vi "Portcullis-CDF State Machine.vi"(0 "Collector Lift State":T1, 1 "Collect Lift Position":dbl, 2 "AutoLift Portcullis?":bool, 3 "AutoAdjust CDF?":bool, 4 "Keep at target?":bool, 5 "See Portcullis?":bool, 6 "See CDF?":bool, 8 "Collector Lift Man.  Request?":bool) -> (20 "Collector Lift State Out":T1)   [LabVIEW 2015]
uses:
  Typedefs/CollectorLiftStates.ctl
panel:
  in  "Thresh":dbl=1.0
  in  "CDF Set Up Position":dbl format="%#_13g"
  in  "Portcullis Set Up Position":dbl format="%#_13g"
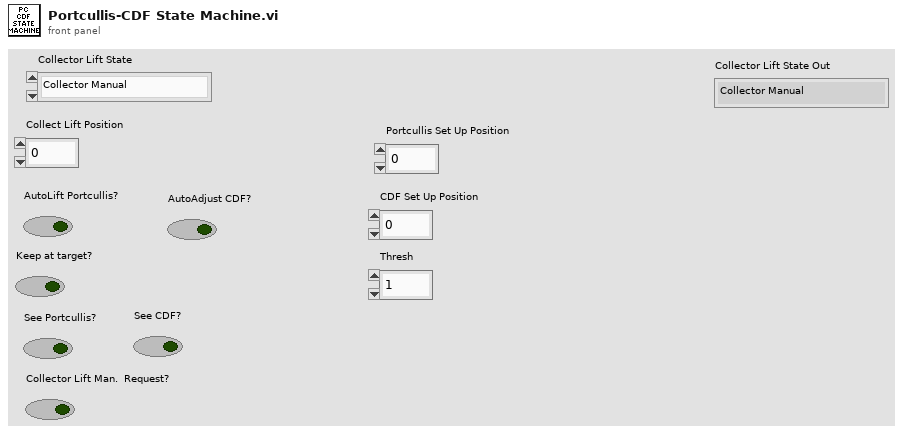
[diagram p1: front panel]
types:
  T1 = typedef "CollectorLiftStates.ctl" = enum16{"Collector Manual", "Stow", "Collect Position", "Spit Position", "Portcullis Set Up", "Portcullis Lift Up", "CDF Set Up", "Push CDF Down"}
  T2 = enum16{"Pass HMI Through Choice", "AutoAdjust CDF", "AutoLift PC"}
  T3 = enum16{"Go to set up ", "Keep at CDF", "Push Down CDF"}
  T4 = enum16{"Go to set up", "Keep At Portcullis", "Lift Up Portcullis"}
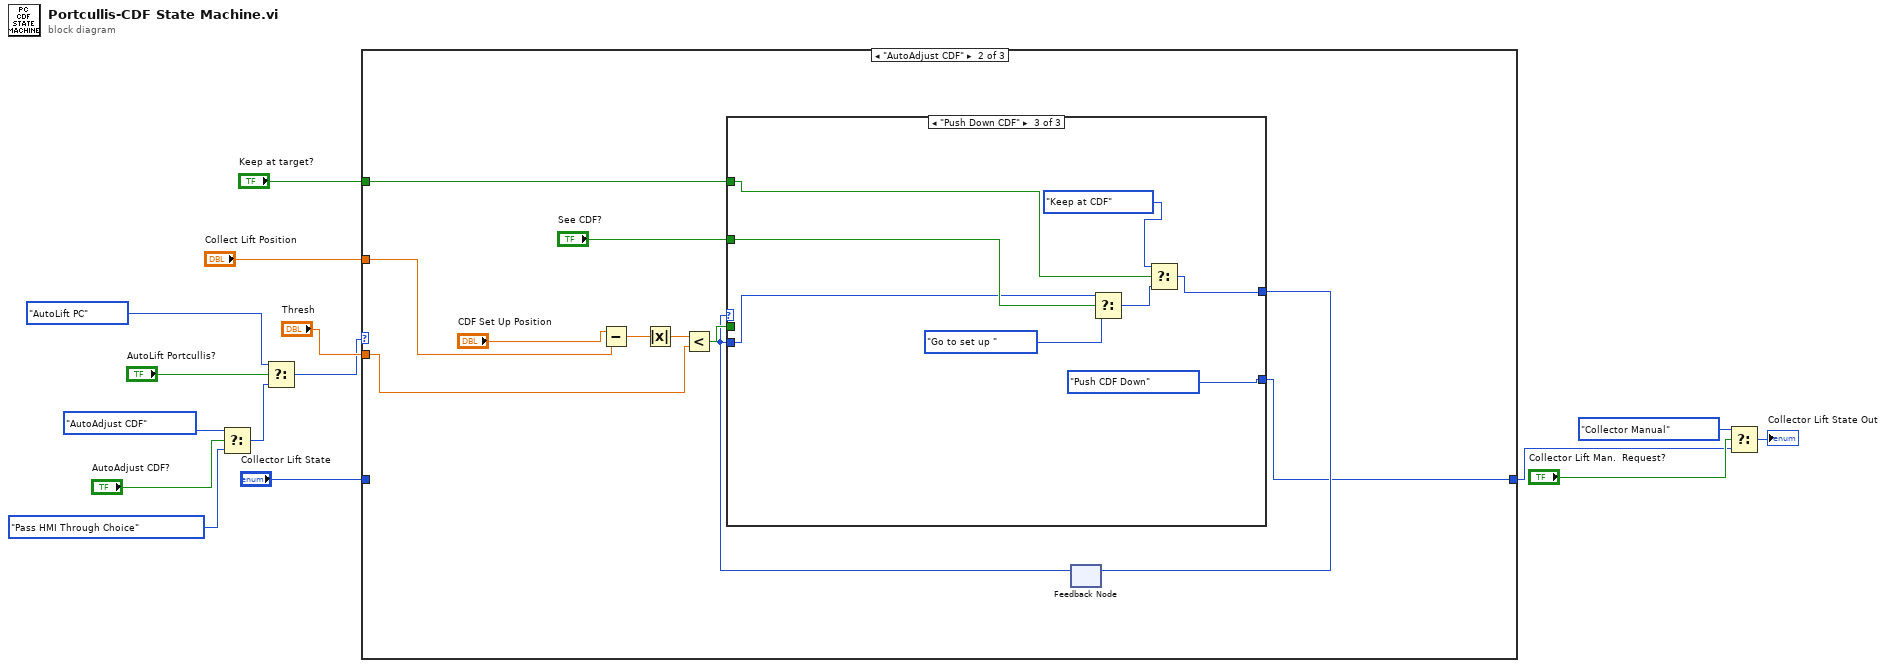
[diagram p0: block diagram]
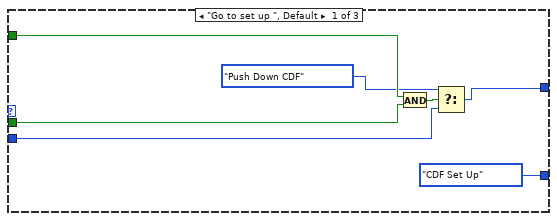
[diagram p3: hidden frame]
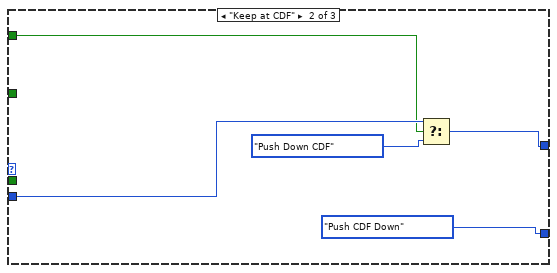
[diagram p4: hidden frame]
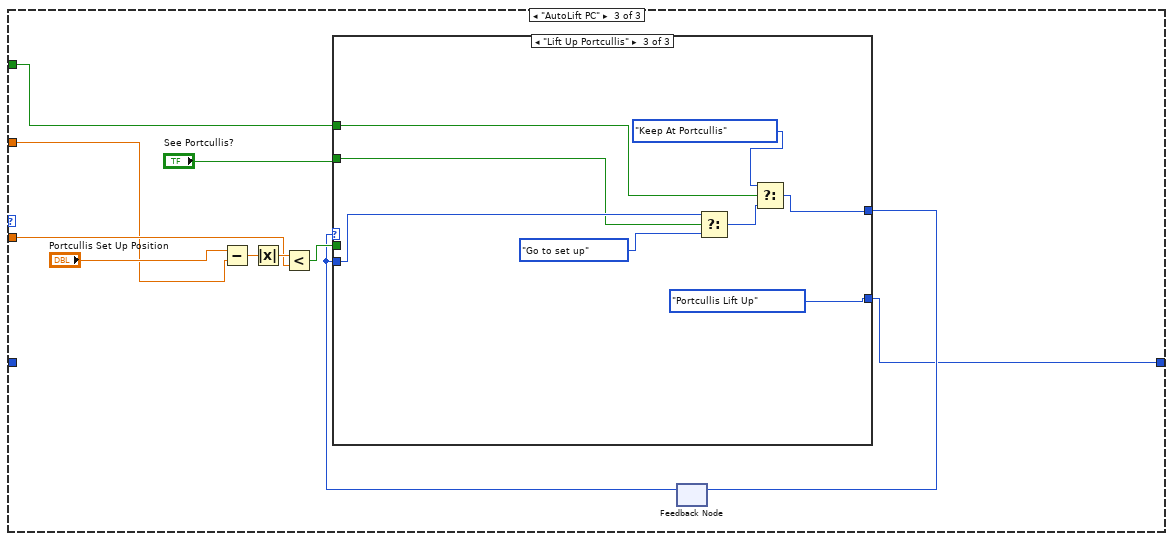
[diagram p5: hidden frame]
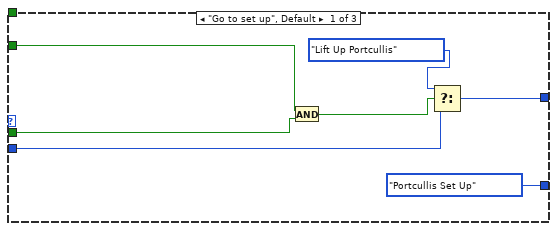
[diagram p6: hidden frame]
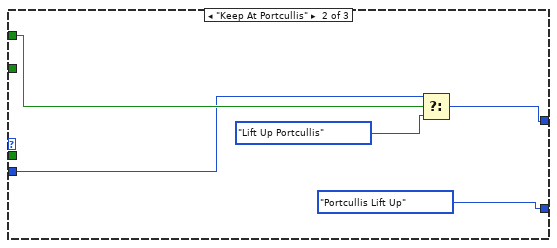
[diagram p7: hidden frame]
diagram:
  n1 = Select(t=T2."AutoAdjust CDF", s="AutoAdjust CDF?", f=T2."Pass HMI Through Choice") -> (s? t:f=w12:T2)
  n2 = Select(t=T2."AutoLift PC", s="AutoLift Portcullis?", f=w12) -> (s? t:f=w5:T2)
  n3 = case shown="\"AutoAdjust CDF\"" w5 {
    tunnel: [w16 w21 w52] -> w3
    tunnel: "Collector Lift State" -> [w16 _ _]
    tunnel: "Collect Lift Position" -> [_ w17 w48]
    tunnel: "Keep at target?" -> [_ w20 w51]
    tunnel: "Thresh" -> [_ w19 w50]
    frame "Pass HMI Through Choice", Default {
      # "Not Going through CDF or Portcullis"
    }
    frame "AutoAdjust CDF" {
      n4 = Subtract(x="CDF Set Up Position", y=w17) -> (x-y=w27:dbl)
      n5 = Absolute Value(x=w27) -> (abs(x)=w26:dbl)
      n6 = Less?(x=w26, y=w19) -> (x < y?=w24:bool)
      n7 = feedback #1() -> (w22:T3)  [unwired: 1 in]
      n8 = case shown="\"Push Down CDF\"" w22 {
        tunnel: [CollectorLiftStates."CDF Set Up" ("Collector Lift States") CollectorLiftStates."Push CDF Down" ("Collector Lift States") CollectorLiftStates."Push CDF Down" ("Collector Lift States")] -> w21
        tunnel: "See CDF?" -> [w33 _ w47]
        tunnel: w24 -> [w32 _ _]
        tunnel: [w30 w38 w45] -> w23
        tunnel: w22 -> [w29 w37 w46]
        tunnel: w20 -> [_ w35 w40]
        frame "Go to set up ", Default {
          n9 = And(x=w33, y=w32) -> (x .and. y?=w31:bool)
          n10 = Select(t=T3."Push Down CDF", s=w31, f=w29) -> (s? t:f=w30:T3)
        }
        frame "Keep at CDF" {
          n11 = Select(t=w37, s=w35, f=T3."Push Down CDF") -> (s? t:f=w38:T3)
        }
        frame "Push Down CDF" {
          n12 = Select(t=w46, s=w47, f=T3."Go to set up ") -> (s? t:f=w44:T3)
          n13 = Select(t=T3."Keep at CDF", s=w40, f=w44) -> (s? t:f=w45:T3)
        }
      }
      n14 = feedback-in #1(w23) -> ()
    }
    frame "AutoLift PC" {
      n15 = Subtract(x="Portcullis Set Up Position", y=w48) -> (x-y=w58:dbl)
      n16 = Absolute Value(x=w58) -> (abs(x)=w57:dbl)
      n17 = Less?(x=w57, y=w50) -> (x < y?=w55:bool)
      n18 = feedback #2() -> (w53:T4)  [unwired: 1 in]
      n19 = case shown="\"Lift Up Portcullis\"" w53 {
        tunnel: [CollectorLiftStates."Portcullis Set Up" ("Collector Lift States") CollectorLiftStates."Portcullis Lift Up" ("Collector Lift States") CollectorLiftStates."Portcullis Lift Up" ("Collector Lift States")] -> w52
        tunnel: "See Portcullis?" -> [w64 _ w71]
        tunnel: w55 -> [w63 _ _]
        tunnel: [w60 w68 w75] -> w54
        tunnel: w53 -> [w59 w66 w77]
        tunnel: w51 -> [_ w69 w74]
        frame "Go to set up", Default {
          n20 = And(x=w64, y=w63) -> (x .and. y?=w61:bool)
          n21 = Select(t=T4."Lift Up Portcullis", s=w61, f=w59) -> (s? t:f=w60:T4)
        }
        frame "Keep At Portcullis" {
          n22 = Select(t=w66, s=w69, f=T4."Lift Up Portcullis") -> (s? t:f=w68:T4)
        }
        frame "Lift Up Portcullis" {
          n23 = Select(t=w77, s=w71, f=T4."Go to set up") -> (s? t:f=w73:T4)
          n24 = Select(t=T4."Keep At Portcullis", s=w74, f=w73) -> (s? t:f=w75:T4)
        }
      }
      n25 = feedback-in #2(w54) -> ()
    }
  }
  n26 = Select(t=CollectorLiftStates."Collector Manual", s="Collector Lift Man.  Request?", f=w3) -> (s? t:f=→"Collector Lift State Out":T1)
